vi "Save_Text_Sequence.vi"(1 "Header":string[](array[string]), 2 "Sequence":cluster{string, string[], dbl[], dbl}[](array[cluster]), 3 "Text File":path) -> ()   [LabVIEW 2011]
doc: "This VI saves the given \"Sequence\" to a text file given by the \"Text File\" parameter. This file can then be loaded back into the growth sequence editor."
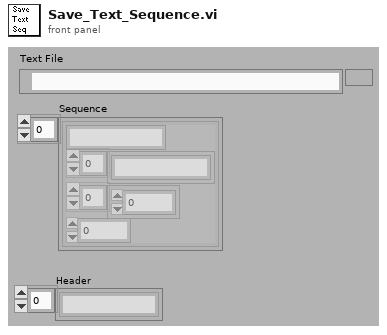
[diagram p1: front panel]
types:
  T1 = cluster{"Command":string, "Header":string[], dbl[], dbl}
  T2 = cluster{"Command":string, "Header":string[], dbl[], dbl}[]
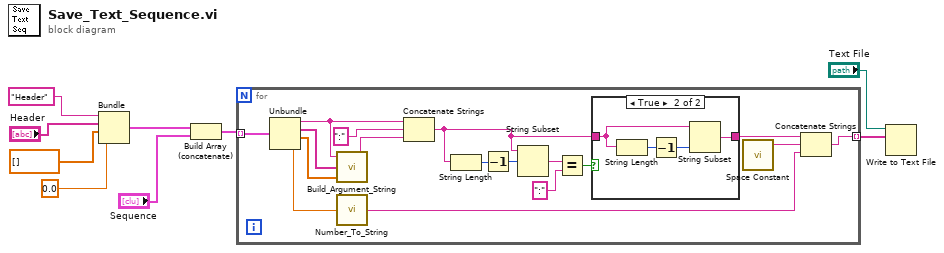
[diagram p0: block diagram]
diagram:
  n1 = Bundle("Command"="Header", "Header"="Header", dbl[] [], 0.0) -> (w4:T1)  [unwired: 1 in]
  n2 = Build Array (concatenate)(w4, "Sequence") -> (w2:T2)
  n3 = for {
    tunnel: w2 -> [w26] mode=indexing
    tunnel: [w13] -> w1 mode=indexing
    n4 = Unbundle(w26) -> ("Command"=w23:string, "Header"=w24:string[], w22:dbl[], w20:dbl)
    n5 = call "Build_Argument_String.vi"("Flow Array"=w22, "Argument List"=w24, "Command"=w23) -> ("Argument String"=w21:string)
    n6 = call "Number_To_String.vi"("Number"=w20) -> ("String"=w10:string)
    n7 = Concatenate Strings(w23, ":" ("string"), w21) -> (w14:string)
    n8 = String Length(string=w14) -> (length=w19:i32)
    n9 = Decrement(x=w19) -> (x-1=w18:i32)
    n10 = String Subset(string=w14, offset (0)=w18) -> (substring=w17:string)  [unwired: 1 out]
    n11 = Equal?(x=w17, y=":") -> (x = y?=w15:bool)
    n12 = case shown="True" w15 {
      tunnel: w14 -> [w27 w29]
      tunnel: [w27 w28] -> w12
      frame False {
      }
      frame True {
        n13 = String Length(string=w29) -> (length=w31:i32)
        n14 = Decrement(x=w31) -> (x-1=w30:i32)
        n15 = String Subset(string=w29, length (rest)=w30) -> (substring=w28:string)  [unwired: 1 in]
      }
    }
    n16 = call <vilib>:"Space Constant.vi"() -> ("String"=w11:string)
    n17 = Concatenate Strings(w12, w11, w10) -> (w13:string)
  }
  n18 = Write to Text File(file (use dialog)="Text File", text=w1) -> ()  [unwired: 1 in, 4 out]
